vi "motorControl.vi"(1 "deceleration":dbl=5.0, 2 "acceleration":dbl=5.0, 3 "velocity":dbl=20.0, 9 "Z":dbl, 10 "Y":dbl, 11 "X":dbl) -> (0 "output cluster":T1)   [LabVIEW 2020]
uses:
  <vilib>/Motion/Express/_s/nimc.ex.straightLineMove.startStraightLineMove.axis.modeRelative.0.vi
  <vilib>/Motion/BlockNode/FB.NIMotion.xnode
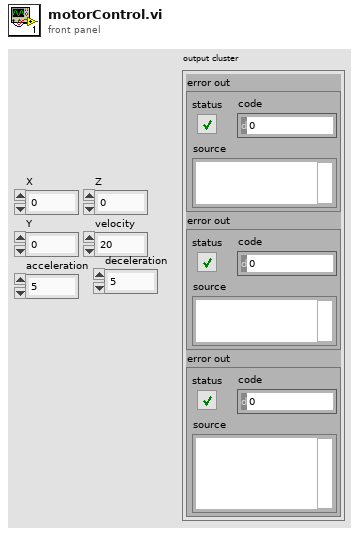
[diagram p1: front panel]
types:
  T1 = cluster{"error out":errorcluster, "error out":errorcluster, "error out":errorcluster}
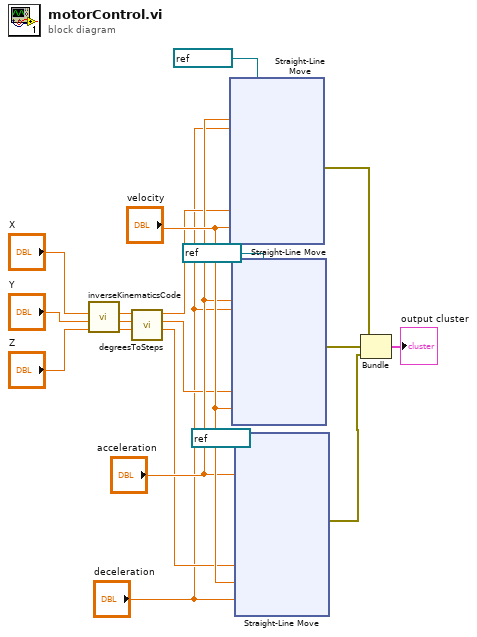
[diagram p0: block diagram]
diagram:
  n1 = call "inverseKinematicsCode.vi"("Z"="Z", "Y"="Y", "X"="X") -> ("THETA3"=w12:dbl, "THETA2"=w13:dbl, "THETA1"=w14:dbl)  [unwired: 6 in]
  n2 = call "degreesToSteps.vi"("theta3"=w12, "theta2"=w13, "theta1"=w14) -> ("steps3"=w9:dbl, "steps2"=w10:dbl, "steps1"=w11:dbl)  [unwired: 6 in]
  n3 = xnode ("Straight-Line Move")("position"=w11, "velocity"="velocity", "resource"=refnum<k21> "Axis 1", "acceleration"="acceleration", "deceleration"="deceleration") -> ("error out"=w5:errorcluster)  [unwired: 5 in, 2 out]
  n4 = xnode ("Straight-Line Move")("position"=w10, "velocity"="velocity", "resource"=refnum<k21> "Axis 2", "acceleration"="acceleration", "deceleration"="deceleration") -> ("error out"=w4:errorcluster)  [unwired: 5 in, 2 out]
  n5 = xnode ("Straight-Line Move")("position"=w9, "velocity"="velocity", "deceleration"="deceleration", "resource"=refnum<k21> "Axis 3", "acceleration"="acceleration") -> ("error out"=w3:errorcluster)  [unwired: 5 in, 2 out]
  n6 = Bundle("error out"=w5, "error out"=w4, "error out"=w3) -> (→"output cluster":T1)  [unwired: 1 in]
